vi "AuMT8852B AFH State.vi"(5 "AFH On? (Off)":bool, 7 "Set/Get (Set)":enum16{"Set", "Get"}(ring)=enum."Get", 8 "error in (no error)":errorcluster, 11 "VISA session":refnum<visa-resource-name>) -> (0 "error out":errorcluster, 2 "error code":i32, 3 "VISA session out":refnum<visa-resource-name>, 4 "AFH On? out":bool)   [LabVIEW 2017]
doc: "Anritsu MT8852B Bluetooth Tester\n\nEnables AFH on the current connection.\nNOTE: Must follow the selection of the display screen.\n\nINPUTS\nSet/Get - whether the value is being sent to or retrieved from the instrument.\nAFH On? - whether to enable AFH on the connection.\n\nOUTPUTS\nAFH On? out - the AFH status on the connection."
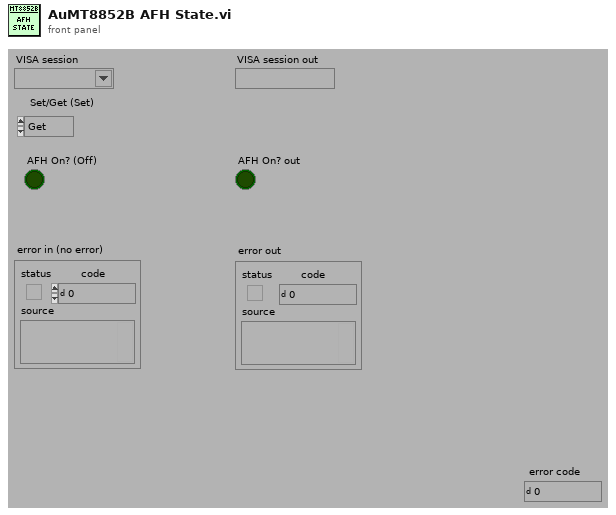
[diagram p1: front panel]
types:
  T1 = enum16{"Simulate", "Range check", "Cache", "Query instrument status"}
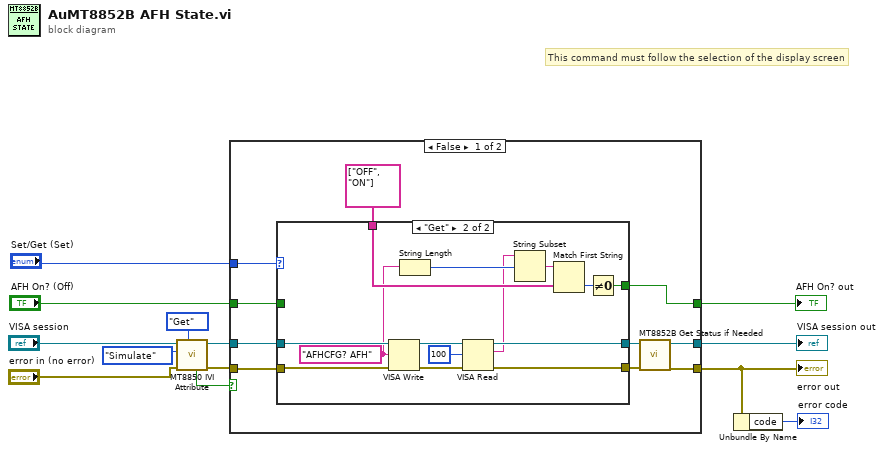
[diagram p0: block diagram]
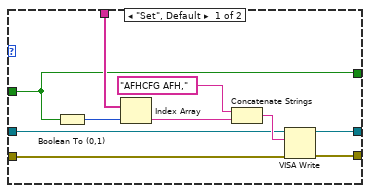
[diagram p2: hidden frame]
diagram:
  # "This command must follow the selection of the display screen"
  n1 = call <instrlib>:"MT8850 IVI Attribute.vi"("Set/Get (Set)"=enum16{"Set", "Get"}."Get", "error in (no error)"="error in (no error)", "Flag (Simulate)"=T1."Simulate", "VISA session"="VISA session") -> ("error out"=w12:errorcluster, "VISA session out"=w13:refnum<visa-resource-name>, "Value out"=w9:bool)  [unwired: 5 in]
  n2 = case shown="False" w9 {
    tunnel: [w19 w50] -> w7
    tunnel: [w20 w49] -> w6
    tunnel: w13 -> [w21 w50]
    tunnel: w12 -> [w22 w49]
    tunnel: [w14 w48] -> w1
    tunnel: "AFH On? (Off)" -> [w16 w48]
    tunnel: "Set/Get (Set)" -> [w15 _]
    frame False {
      n3 = case shown="\"Get\"" w15 {
        tunnel: string[] ["OFF", "ON"] -> [w33 w44]
        tunnel: w16 -> [w24 _]
        tunnel: [w24 w38] -> w14
        tunnel: [w26 w41] -> w17
        tunnel: [w27 w40] -> w18
        tunnel: w22 -> [w29 w43]
        tunnel: w21 -> [w28 w42]
        frame "Set", Default {
          n4 = Boolean To (0,1)(Boolean=w24) -> (0, 1=w25:i16)
          n5 = Index Array(array=w33, index=w25) -> (element=w32:string)
          n6 = Concatenate Strings("AFHCFG AFH," ("write buffer (\"\")"), w32) -> (w30:string)
          n7 = VISA Write(VISA resource name=w28, write buffer=w30, error in (no error)=w29) -> (VISA resource name out=w27:refnum<visa-resource-name>, error out=w26:errorcluster)  [unwired: 1 out]
        }
        frame "Get" {
          w35 = "AFHCFG? AFH" ("write buffer (\"\")")
          n8 = VISA Write(VISA resource name=w42, write buffer=w35, error in (no error)=w43) -> (VISA resource name out=w46:refnum<visa-resource-name>, error out=w47:errorcluster)  [unwired: 1 out]
          n9 = String Length(string=w35) -> (length=w36:i32)
          n10 = VISA Read(VISA resource name=w46, byte count=u32 100 ("byte count (0)"), error in (no error)=w47) -> (VISA resource name out=w40:refnum<visa-resource-name>, read buffer=w34:string, error out=w41:errorcluster)  [unwired: 1 out]
          n11 = String Subset(string=w34, offset (0)=w36) -> (substring=w37:string)  [unwired: 1 in]
          n12 = Match First String(2:w44, 3:w37) -> (0:w39:i32)  [unwired: 1 out]
          n13 = Not Equal To 0?(x=w39) -> (x != 0?=w38:bool)
        }
      }
      n14 = call <instrlib>:"MT8852B Get Status if Needed.vi"("error in (no error)"=w17, "VISA session"=w18) -> ("error out"=w20:errorcluster, "VISA session out"=w19:refnum<visa-resource-name>)  [unwired: 8 in]
    }
    frame True {
    }
  }
  "error out" <- w6
  "VISA session out" <- w7
  "AFH On? out" <- w1
  n15 = Unbundle By Name(w6) -> ("code"=→"error code":i32)
